vi "Async Bus Load Calculator.vi"(8 "error in (no error)":errorcluster, 10 "Comm Queues":T1, 11 "Calculation Period (ms)":u32) -> (0 "error out":errorcluster)   [LabVIEW 2019, in "XNET-Bus-Load-Calculator.lvlib" / "GenBus_Load_Calculator.lvclass"]
uses:
  GenBus_Load_Calculator.lvclass
  typedefs/Calc_Comm_Refs.ctl
  typedefs/ToCalculator_Data.ctl
  typedefs/FromCalculator_Data.ctl
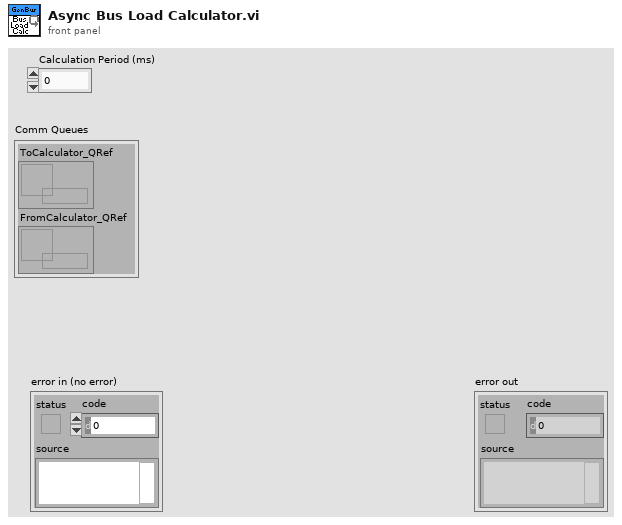
[diagram p1: front panel]
types:
  T1 = typedef "XNET-Bus-Load-Calculator.lvlib/GenBus_Load_Calculator.lvclass/Calc_Comm_Refs.ctl" = cluster{"ToCalculator_QRef":refnum<queue>, "FromCalculator_QRef":refnum<queue>}
  T2 = typedef "XNET-Bus-Load-Calculator.lvlib/GenBus_Load_Calculator.lvclass/FromCalculator_Data.ctl" = cluster{"Bus Load (%)":dbl}
  T3 = typedef "XNET-Bus-Load-Calculator.lvlib/GenBus_Load_Calculator.lvclass/ToCalculator_Data.ctl" = cluster{"Stop":bool, "Bus Busy Time (us)":u64}
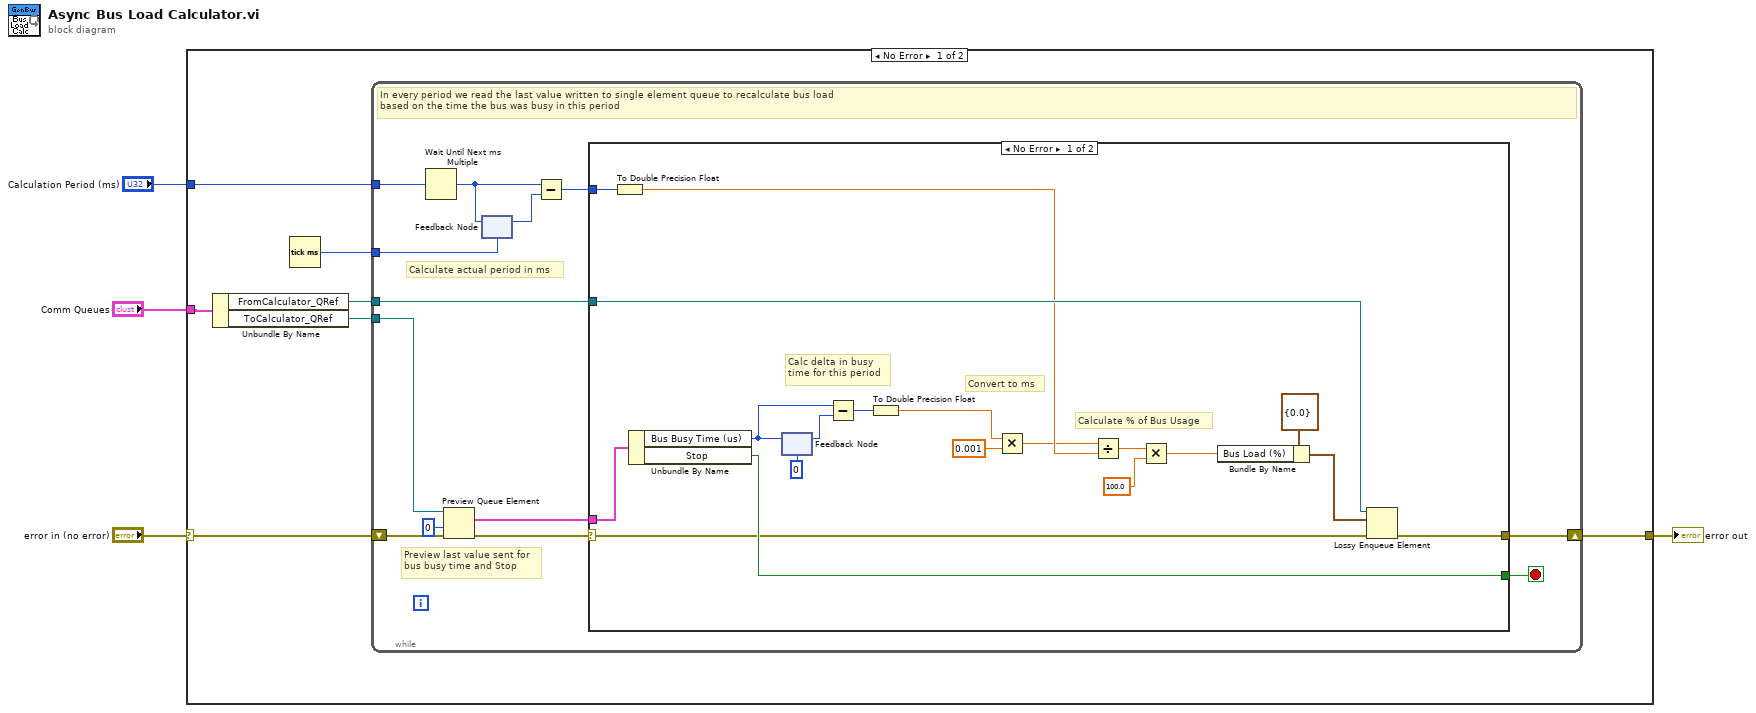
[diagram p0: block diagram]
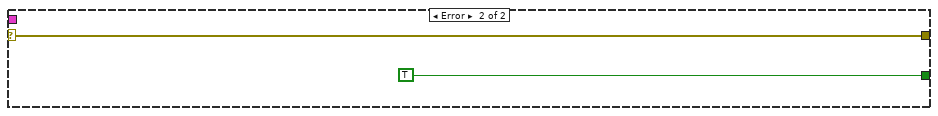
[diagram p2: hidden frame]
diagram:
  n1 = case shown="No Error" "error in (no error)" {
    selector: "error in (no error)" -> [w11 w46]
    tunnel: [w7 w46] -> w3
    tunnel: "Comm Queues" -> [w10 _]
    tunnel: "Calculation Period (ms)" -> [w8 _]
    frame No Error {
      n2 = Unbundle By Name(w10) -> ("FromCalculator_QRef"=w5:refnum<queue>, "ToCalculator_QRef"=w9:refnum<queue>)
      n3 = Tick Count (ms)() -> (millisecond timer value=w6:u32)
      n4 = while {
        tunnel: w9 -> [w23]
        tunnel: w8 -> [w20]
        tunnel: w6 -> [w13]
        shift-right: [w17] -> w7
        shift-left: w11 -> [w24]
        tunnel: w5 -> [w12]
        stop <- w18 stop-if-true
        # "Preview last value sent for\nbus busy time and Stop"
        # "Calculate actual period in ms"
        # "In every period we read the last value written to single element queue to recalculate bus load\nbased on the time the bus was busy in this period"
        n5 = Wait Until Next ms Multiple(millisecond multiple=w20) -> (millisecond timer value=w15:u32)
        n6 = Preview Queue Element(queue=w23, timeout in ms (-1)=0, error in (no error)=w24) -> (element=w19:T3, error out=w22:errorcluster)  [unwired: 2 out]
        n7 = feedback-in #1(w15) -> ()
        n8 = feedback #1(w13) -> (w16:u32)
        n9 = Subtract(x=w15, y=w16) -> (x-y=w14:u32)
        n10 = case shown="No Error" w22 {
          selector: w22 -> [w38 w44]
          tunnel: w19 -> [w43 _]
          tunnel: [w42 TRUE] -> w18
          tunnel: [w40 w44] -> w17
          tunnel: w14 -> [w41 _]
          tunnel: w12 -> [w39 _]
          frame No Error {
            # "Calc delta in busy\ntime for this period"
            # "Calculate % of Bus Usage"
            # "Convert to ms"
            n11 = To Double Precision Float(number=w41) -> (double precision float=w34:dbl)
            n12 = Unbundle By Name(w43) -> ("Bus Busy Time (us)"=w29:u64, "Stop"=w42:bool)
            n13 = feedback-in #2(w29) -> ()
            n14 = feedback #2(u64 0 ("Bus Busy Time (us)")) -> (w28:u64)
            n15 = Subtract(x=w29, y=w28) -> (x-y=w26:u64)
            n16 = To Double Precision Float(number=w26) -> (double precision float=w25:dbl)
            n17 = Multiply(x=w25, y=0.001) -> (x*y=w32:dbl)
            n18 = Divide(x=w32, y=w34) -> (x/y=w31:dbl)
            n19 = Multiply(x=w31, y=100.0) -> (x*y=w36:dbl)
            n20 = Bundle By Name(cluster=T2 {"Bus Load (%)"=0.0} ("FromCalculator_Data"), "Bus Load (%)"=w36) -> (w35:T2)
            n21 = Lossy Enqueue Element(queue=w39, element=w35, error in (no error)=w38) -> (error out=w40:errorcluster)  [unwired: 3 out]
          }
          frame Error {
          }
        }
      }
    }
    frame Error {
    }
  }
  "error out" <- w3
